vi "signal generator.vi"() -> ()   [LabVIEW 2012]
panel:
  out "Waveform Graph 2":dynamicdata(graph)
  out "Waveform Graph":dynamicdata(graph)
  in  "stop":bool
  out "Scan Signal":cluster{"Y":dbl[], "Y":dbl[]}[](graph)
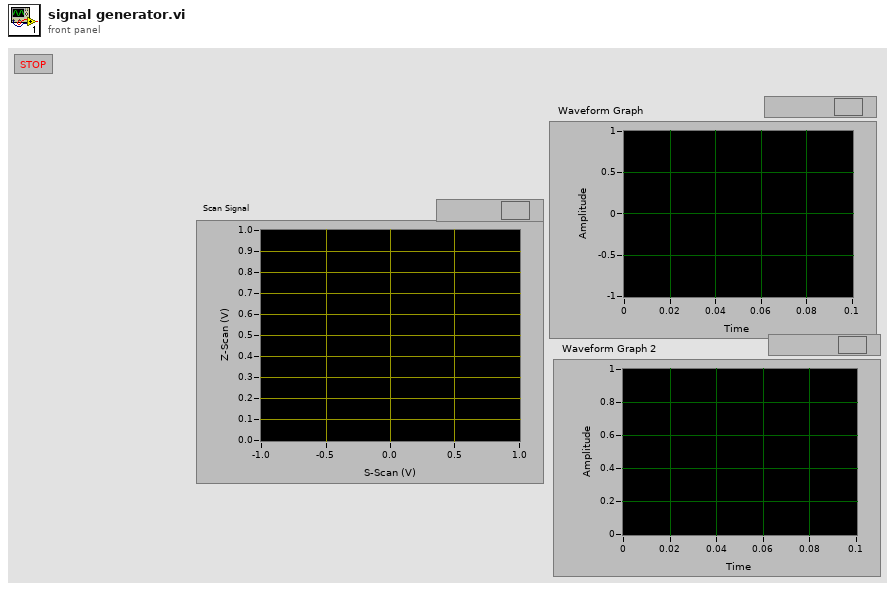
[diagram p1: front panel]
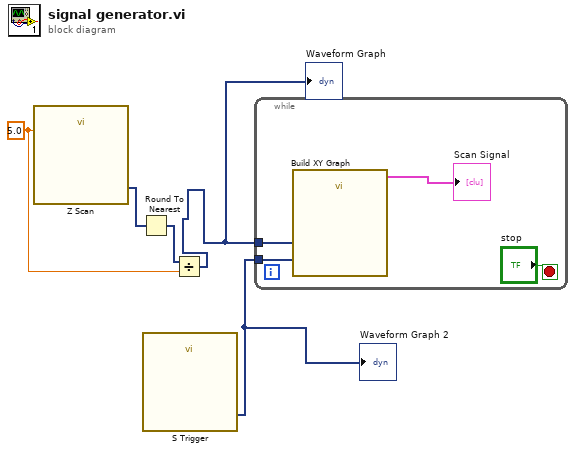
[diagram p0: block diagram]
diagram:
  w1 = 5.0 ("Amplitude")
  n1 = call "Z Scan"("Amplitude"=w1) -> ("Triangle"=w4:dynamicdata)  [unwired: 13 in, 1 out]
  n2 = Round To Nearest(number=w4) -> (nearest integer value=w3:dynamicdata)
  n3 = call "S Trigger"() -> ("Triangle"=w5:dynamicdata)  [unwired: 14 in, 1 out]
  "Waveform Graph 2" <- w5
  n4 = Divide(x=w3, y=w1) -> (x/y=w2:dynamicdata)
  "Waveform Graph" <- w2
  n5 = while {
    tunnel: w2 -> [w8]
    tunnel: w5 -> [w7]
    stop <- "stop" stop-if-true
    n6 = call "Build XY Graph"("Y Input"=w7, "X Input"=w8) -> ("XY Graph"=→"Scan Signal":cluster{"Y":dbl[], "Y":dbl[]}[])  [unwired: 3 in, 6 out]
  }
